vi "MM6Archiver.compile DAQ data.vi"(0 "i ref in":refnum<vi>, 1 "timeStamp":dbl, 2 "eventData":T1, 5 "error in (no error)":errorcluster) -> (14 "i ref out":refnum<vi>, 16 "trapData":string, 19 "error out":errorcluster)   [LabVIEW 2014, in "MM6Archiver.lvlib"]
doc: "Analyzes the DAQ data assuming that the first device is a multi channel scaler producing time-of-flight data in waveform format. Then it compiles the data into the format used MM6 and EVA."
uses:
  MM6Archiver.lvlib
  CSCore/CSSystem/CoreDefs/CoreDefs.rawDataType.ctl
  CSCore/CSSystem/CoreDefs/CoreDefs.error_severity.ctl
  CSCore/CSSystem/CoreDefs/CoreDefs.error_type.ctl
  CSCore/CSSystem/CoreLib/CoreLib.byte array 2 double.vi
  CSCore/CSSystem/CoreLib/CoreLib.byte array 2 double array.vi
  CSData/DataLib/DataLib.lvlib
  CSCore/CSSystem/CoreLib/CoreLib.lvlib
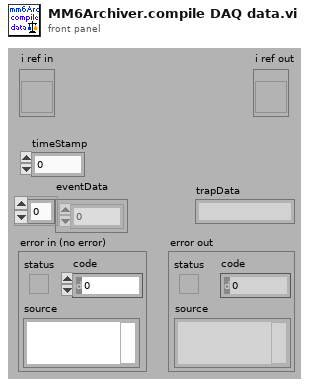
[diagram p1: front panel]
types:
  T1 = typedef "CoreDefs.rawDataType.ctl" = i8[]
  T2 = typedef "CoreDefs.error_type.ctl" = enum16{"no error", "can't load process", "can't unload process", "process does not exist", "can't install process", "can't remove process", "unknown function", "time out", "can't execute function", "duplicate queue name", "super not found", "caller queue invalid", "can't ping process", "unknown error", "VISA Error", "VISA timeout", "GPIB timeout", "GPIB error", "communication error", "data type mismatch", "can't read data from OPC server", "can't write data to OPC server", "OET error", "function not implemented", "process already exists", "invalid Shared Variable name", "error writing Shared Variable", "error reading Shared Variable", "invalid client name", "corrupt database", "unknown class", "call not authorized", "parameter out of range", "OET timeout: can't get data to modify", "invalid queue name", "requested operation incompatible with current state", "event undefined", "event disabled", "state undefined", "caller is not a friend", "EventBuilder: bad eventID", "EventBuilder: no DAQ devices", "a thread must not stop itself", "UNUSED ELEMENT4", "DiscArchiver: eventData incomplete", "DiscArchiver: eventData does not belong to run", "DiscArchiver: can't open file", "DiscArchiver: can't write to file", "DiscArchiver: available disc space low", "can't acquire semaphore", "error reading data from database", "notifier object is not existing", "can't register process", "can't unregister process", "illegal event type", "object disabled", "object already exists", "can't change state", "Instrument not found", "no connection to remote node", "invalid reference", "N/A", "UNUSED ELEMENT 1", "element not found", "illegal TCP/IP connection detected", "object does not exist", "invalid access ID", "unknown CS system", "invalid privilige", "unsupported data type", "unsupported server type", "IO server already exists", "Shared Variable already exists"}
  T3 = typedef "CoreDefs.error_severity.ctl" = enum16{"undefined", "information", "warning", "error", "fatal"}
  T4 = typedef "BaseProcess.lvlib/BaseProcess.descriptor string definition.ctl" = string
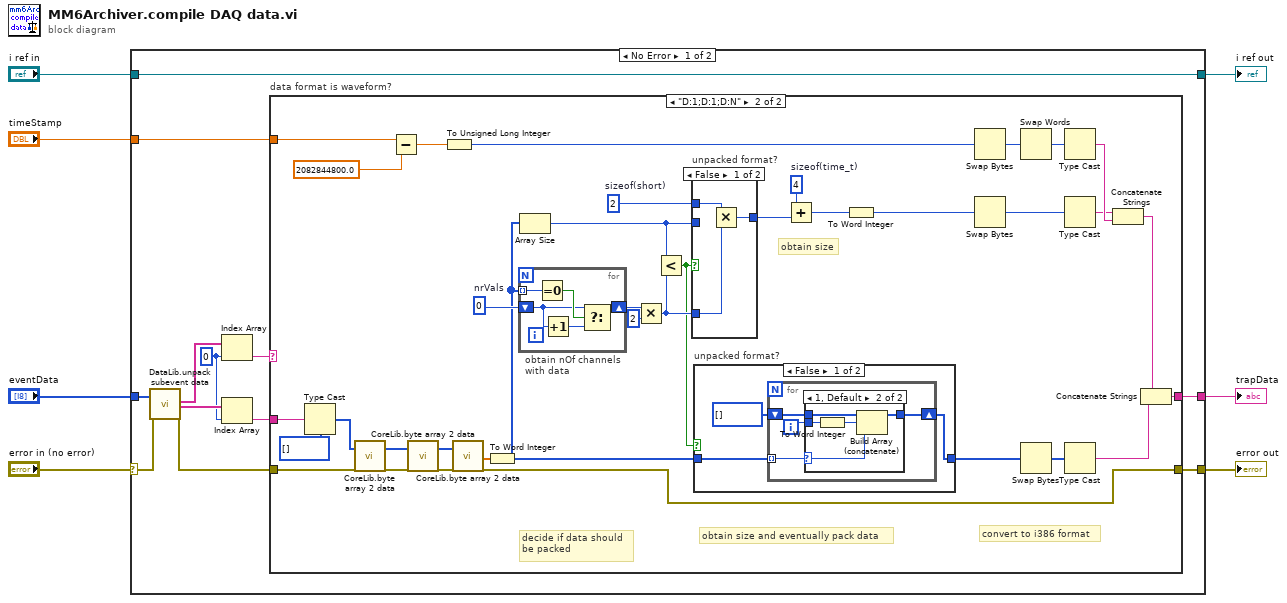
[diagram p0: block diagram]
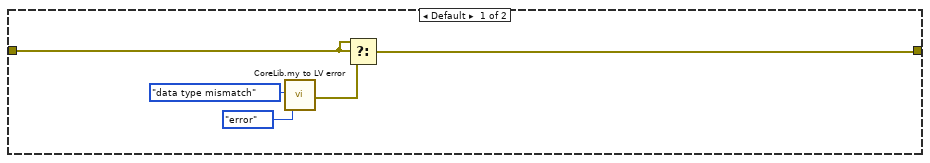
[diagram p2: hidden frame]
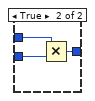
[diagram p5: hidden frame]
diagram:
  n1 = case shown="No Error" "error in (no error)" {
    selector: "error in (no error)" -> [w17 w86]
    tunnel: "i ref in" -> [w19 w87]
    tunnel: [w19 w87] -> w6
    tunnel: [w12 w86] -> w5
    tunnel: "eventData" -> [w18 _]
    tunnel: [w9 _] -> w2
    tunnel: "timeStamp" -> [w8 _]
    frame No Error {
      w14 = 0 ("index")
      n2 = call "DataLib.unpack subevent data.vi"("subeventData"=w18, "error in (no error)"=w17) -> ("dataDescriptors"=w16:T4[], "subeventData"=w15:string[], "error out"=w11:errorcluster)  [unwired: 14 in, 1 out]
      n3 = Index Array(array=w16, index=w14) -> (element=w13:T4)
      n4 = Index Array(array=w15, index=w14) -> (element=w10:string)
      n5 = case "data format is waveform?" shown="\"D:1;D:1;D:N\"" w13 {
        tunnel: [w22 w31] -> w12
        tunnel: w11 -> [w20 w55]
        tunnel: w10 -> [_ w56]
        tunnel: [_ w32] -> w9
        tunnel: w8 -> [_ w28]
        frame Default {
          n6 = call "CoreLib.my to LV error.vi"("ErrorTypes"=CoreDefs.error_type."data type mismatch", "severityLevel"=CoreDefs.error_severity."error") -> ("myErrorCluster"=w21:errorcluster)  [unwired: 16 in, 1 out]
          n7 = Select(t=w20, s=w20, f=w21) -> (s? t:f=w22:errorcluster)
        }
        frame "D:1;D:1;D:N" {
          w47 = 2  # sizeof(short)
          w45 = 4  # sizeof(time_t)
          w51 = 0  # nrVals
          # "convert to i386 format"
          # "obtain size"
          # "obtain size and eventually pack data"
          # "decide if data should\nbe packed"
          n8 = Type Cast(type=T1 [] ("Array"), x=w56) -> (*(type *) &x=w60:T1)
          n9 = call-poly "CoreLib.byte array 2 data.vi"("byteArray"=w60, "error in (no error)"=w55) -> ("byteArray out"=w58:T1, "error out"=w54:errorcluster)  [unwired: 15 in, 1 out]
          n10 = Subtract(x=w28, y=2082844800.0 ("x-y")) -> (x-y=w26:dbl)
          n11 = call-poly "CoreLib.byte array 2 data.vi"("byteArray"=w58, "error in (no error)"=w54) -> ("byteArray out"=w57:T1, "error out"=w53:errorcluster)  [unwired: 15 in, 1 out]
          n12 = To Unsigned Long Integer(number=w26) -> (unsigned 32bit integer=w25:u32)
          n13 = call-poly "CoreLib.byte array 2 data.vi"("byteArray"=w57, "error in (no error)"=w53) -> ("[d64]"=w52:dbl[], "error out"=w31:errorcluster)  [unwired: 15 in, 1 out]
          n14 = To Word Integer(number=w52) -> (16bit integer=w41:i16[])
          n15 = for "obtain nOf channels\nwith data" {
            tunnel: w41 -> [w85] mode=indexing
            shift-right: [w81] -> w50
            shift-left: w51 -> [w83]
            n16 = Equal To 0?(x=w85) -> (x = 0?=w84:bool)
            n17 = Increment(x=w83) -> (x+1=w82:i32)
            n18 = Select(t=w83, s=w84, f=w82) -> (s? t:f=w81:i32)
          }
          n19 = Array Size(array=w41) -> (size(s)=w48:i32)
          n20 = Multiply(x=w50, y=2) -> (x*y=w44:i32)
          n21 = Less?(x=w48, y=w44) -> (x < y?=w42:bool)
          n22 = case "unpacked format?" shown="False" w42 {
            tunnel: w48 -> [_ w80]
            tunnel: w47 -> [w77 w79]
            tunnel: [w75 w78] -> w46
            tunnel: w44 -> [w76 _]
            frame False {
              n23 = Multiply(x=w77, y=w76) -> (x*y=w75:i32)
            }
            frame True {
              n24 = Multiply(x=w79, y=w80) -> (x*y=w78:i32)
            }
          }
          n25 = case "unpacked format?" shown="False" w42 {
            tunnel: w41 -> [w63 w74]
            tunnel: [w61 w74] -> w36
            frame False {
              n26 = for {
                tunnel: w63 -> [w67] mode=indexing
                shift-right: [w65] -> w61
                shift-left: i16[] [] -> [w66]
                i -> [w64]
                n27 = case shown="1, Default" w67 {
                  selector: w67 -> [_ w70]
                  tunnel: w66 -> [w68 w73]
                  tunnel: [w68 w72] -> w65
                  tunnel: w64 -> [_ w71]
                  frame 0 {
                  }
                  frame 1, Default {
                    n28 = To Word Integer(number=w71) -> (16bit integer=w69:i16)
                    n29 = Build Array (concatenate)(w73, w69, w70) -> (w72:i16[])
                  }
                }
              }
            }
            frame True {
            }
          }
          n30 = Add(x=w45, y=w46) -> (x+y=w43:i32)
          n31 = To Word Integer(number=w43) -> (16bit integer=w30:i16)
          n32 = Swap Bytes(anything=w25) -> (byte swapped=w39:u32)
          n33 = Swap Bytes(anything=w30) -> (byte swapped=w29:i16)
          n34 = Swap Words(1:w39) -> (0:w40:u32)
          n35 = Swap Bytes(anything=w36) -> (byte swapped=w37:i16[])
          n36 = Type Cast(x=w40) -> (*(type *) &x=w38:string)  [unwired: 1 in]
          n37 = Type Cast(x=w29) -> (*(type *) &x=w35:string)  [unwired: 1 in]
          n38 = Type Cast(x=w37) -> (*(type *) &x=w34:string)  [unwired: 1 in]
          n39 = Concatenate Strings(w35, w38) -> (w33:string)
          n40 = Concatenate Strings(w33, w34) -> (w32:string)
        }
      }
    }
    frame Error {
    }
  }
  "error out" <- w5
  "i ref out" <- w6
  "trapData" <- w2
